vi "Chroma_19020_Start.vi"(8 "error in (no error)":errorcluster caption="错误输入（无错误）", 11 "VISA引用句柄输入":refnum<visa-resource-name>) -> (0 "error out":errorcluster caption="错误输出", 3 "VISA引用句柄输出":refnum<visa-resource-name>)   [LabVIEW 2018]
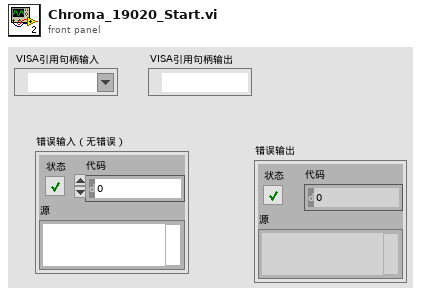
[diagram p1: front panel]
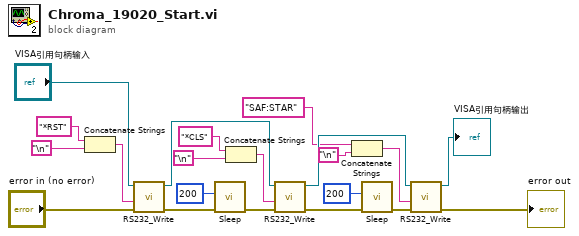
[diagram p0: block diagram]
diagram:
  n1 = Concatenate Strings("*RST" ("写入缓冲区"), "\n") -> (w14:string)
  n2 = call "RS232_Write.vi"("错误输入（无错误）"="error in (no error)", "写入缓冲区"=w14, "VISA资源名称"="VISA引用句柄输入") -> ("错误输出"=w19:errorcluster, "VISA资源名称输出"=w18:refnum<visa-resource-name>)  [unwired: 7 in]
  n3 = call "Sleep.vi"("error in (no error)"=w19, "等待时间（毫秒）"=u32 200) -> ("error out"=w21:errorcluster)  [unwired: 9 in]
  n4 = Concatenate Strings("*CLS" ("写入缓冲区"), "\n") -> (w17:string)
  n5 = call "RS232_Write.vi"("错误输入（无错误）"=w21, "写入缓冲区"=w17, "VISA资源名称"=w18) -> ("错误输出"=w9:errorcluster, "VISA资源名称输出"=w5:refnum<visa-resource-name>)  [unwired: 7 in]
  n6 = Concatenate Strings("SAF:STAR" ("写入缓冲区"), "\n") -> (w6:string)
  n7 = call "Sleep.vi"("error in (no error)"=w9, "等待时间（毫秒）"=u32 200) -> ("error out"=w10:errorcluster)  [unwired: 9 in]
  n8 = call "RS232_Write.vi"("错误输入（无错误）"=w10, "写入缓冲区"=w6, "VISA资源名称"=w5) -> ("错误输出"=→"error out":errorcluster, "VISA资源名称输出"=→"VISA引用句柄输出":refnum<visa-resource-name>)  [unwired: 7 in]
